vi "MVP Valve Initialize.vi"(0 "VISA resource name":refnum<visa-resource-name>="VALVE", 9 "Baud Rate (9600)":u32(ring)=9600 items=["300"=300, "1200"=1200, "2400"=2400, "9600"=9600], 11 "error in (no error)":errorcluster) -> (4 "VISA resource name out":refnum<visa-resource-name>, 15 "error out":errorcluster)   [LabVIEW 2015]
doc: "This VI passes the addressing information in the instrument decriptor to the Instr Open VI and returns the instrument ID. You must run this VI before using any of the instrument driver VIs for this instrument.\n\nNote:\nOnly one Initialize.vi is required when programming multiple instruments on the same port."
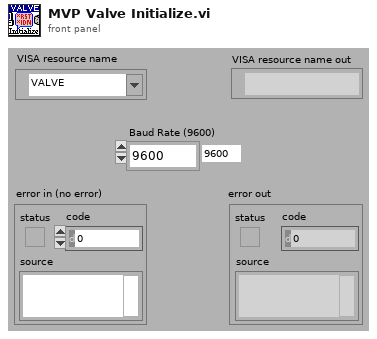
[diagram p1: front panel]
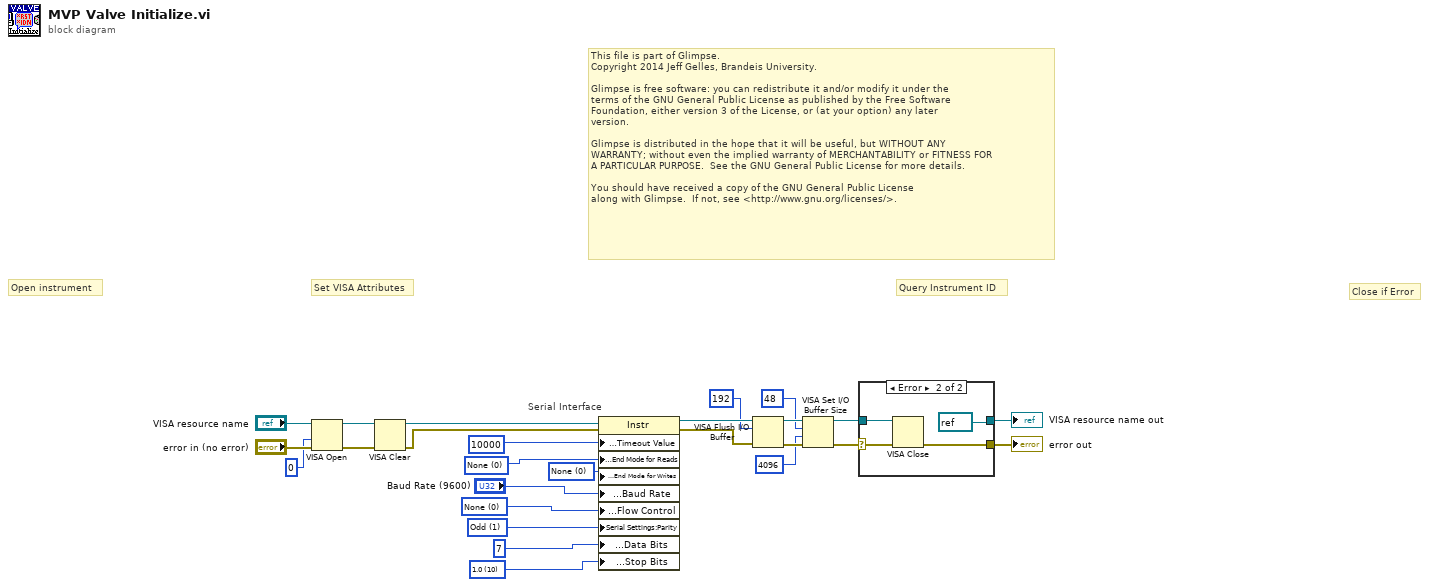
[diagram p0: block diagram]
diagram:
  w3 = u16 10 items=["1.0"=10, "1.5"=15, "2.0"=20] ("Serial Settings:Serial Stop Bits")
  w5 = u16 1 items=["None", "Odd", "Even", "Mark", "Space"] ("Serial Settings:Serial Parity")
  w6 = u16 0 items=["None"=0, "XON/XOFF"=1, "RTS/CTS"=2, "DTR/DSR"=4, "XON/XOFF & RTS/CTS"=3, "XON/XOFF & DTR/DSR"=5] ("Serial Settings:Serial Flow Control")
  w8 = u16 0 items=["None", "LastBit", "TermChar", "Break"] ("Serial Settings:Serial End Mode for Writes")
  w12 = u16 0 items=["None", "LastBit", "TermChar"] ("Serial Settings:Serial End Mode for Reads")
  # "This file is part of Glimpse. \nCopyright 2014 Jeff Gelles, Brandeis University.    \n\nGlimpse is free software: you can redistribute it and/or modify it under the \nterms of the GNU General Public License as published by the Free Software \nFoundation, either version 3 of the License, or (at your option) any later \nversion.\n\nGlimpse is distributed in the hope that it will be useful, but WITHOUT ANY \nWARRANTY; without even the implied warranty of MERCHANTABILITY or FITNESS FOR \nA PARTICULAR PURPOSE.  See the GNU General Public License for more details.\n\nYou should have received a copy of the GNU General Public License\nalong with Glimpse.  If not, see <http://www.gnu.org/licenses/>."
  # "Serial Interface"
  # "Set VISA Attributes"
  # "Close if Error"
  # "Query Instrument ID"
  # "Open instrument"
  n1 = VISA Open(access mode=u32 0, error in (no error)="error in (no error)", VISA resource name="VISA resource name") -> (VISA resource name=w21:refnum<visa-resource-name>, error out=w20:errorcluster)  [unwired: 2 out]
  n2 = VISA Clear(VISA resource name=w21, error in (no error)=w20) -> (VISA resource name out=w10:refnum<visa-resource-name>, error out=w9:errorcluster)
  n3 = property class="Instr"(reference=w10, error in=w9, "General Settings:Timeout Value"=u32 10000, "Serial Settings:End Mode for Reads"=w12, "Serial Settings:End Mode for Writes"=w8, "Serial Settings:Baud Rate"="Baud Rate (9600)", "Serial Settings:Flow Control"=w6, "Serial Settings:Parity"=w5, "Serial Settings:Data Bits"=u16 7 ("Serial Settings:Serial Data Bits"), "Serial Settings:Stop Bits"=w3) -> (reference out=w16:refnum<visa-resource-name>, error out=w18:errorcluster)
  n4 = VISA Flush I/O Buffer(VISA resource name=w16, mask (16)=u16 192, error in (no error)=w18) -> (VISA resource name out=w19:refnum<visa-resource-name>, error out=w17:errorcluster)
  n5 = VISA Set I/O Buffer Size(VISA resource name=w19, mask (16)=u16 48, size (4096)=u32 4096 ("size (0)"), error in (no error)=w17) -> (VISA resource name out=w2:refnum<visa-resource-name>, error out=w1:errorcluster)
  n6 = case shown="Error" w1 {
    selector: w1 -> [w27 w30]
    tunnel: w2 -> [w28 w31]
    tunnel: [w28 refnum<visa-resource-name> refnum ("VISA resource name")] -> w26
    tunnel: [w27 w32] -> w25
    frame No Error {
    }
    frame Error {
      n7 = VISA Close(VISA resource name=w31, error in (no error)=w30) -> (error out=w32:errorcluster)
    }
  }
  "VISA resource name out" <- w26
  "error out" <- w25
